vi "Linear Fit (LS).vi"(0 "Y":dbl[](array[numeric]) format="%#.6g", 5 "X":dbl[](array[numeric]) format="%#.6g", 7 "Weight":dbl[](array[numeric]) format="%#.6g") -> (4 "Best Linear Fit":dbl[](array[numeric]) format="%#.6g", 6 "slope":dbl format="%#.6g", 8 "intercept":dbl format="%#.6g", 14 "residue":dbl format="%#.6g", 15 "error":i32)   [LabVIEW 2020, in "NI_AALPro.lvlib"]
uses:
  <vilib>/Analysis/NI_AALPro.lvlib
  <resource>/lvanlys.dll
panel:
  # "LS Linear Fit"
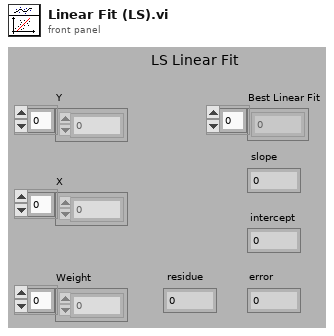
[diagram p1: front panel]
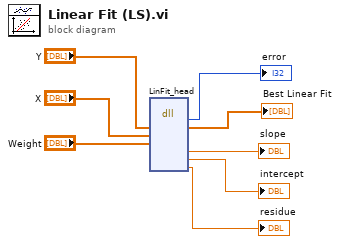
[diagram p0: block diagram]
diagram:
  n1 = dll-call lib="e:/builds/penguin/labview/branches/2020/dev/dist/resource/lvanlys.*" fn="LinFit_head"("yH"="Y", "xH"="X", "weightH"="Weight") -> (→"error":i32, "yH"=→"Best Linear Fit":dbl[], "slope"=→"slope":dbl, "intercept"=→"intercept":dbl, "meanErr"=→"residue":dbl)  [unwired: 8 in, 2 out]
